vi "数据库插入子vi.vi"(2 "result":string, 3 "2_Leakage":string, 8 "2_Pressure":string, 10 "Serial_No":string) -> ()   [LabVIEW 2014]
panel:
  out "error out":errorcluster
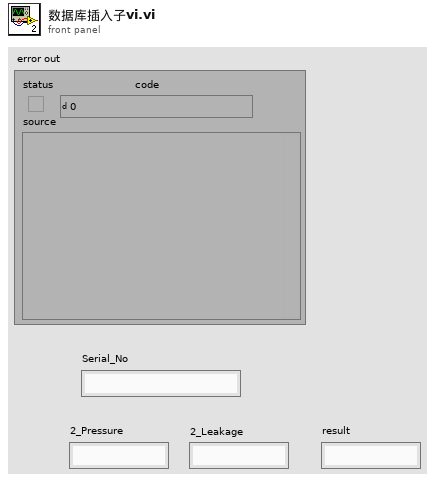
[diagram p1: front panel]
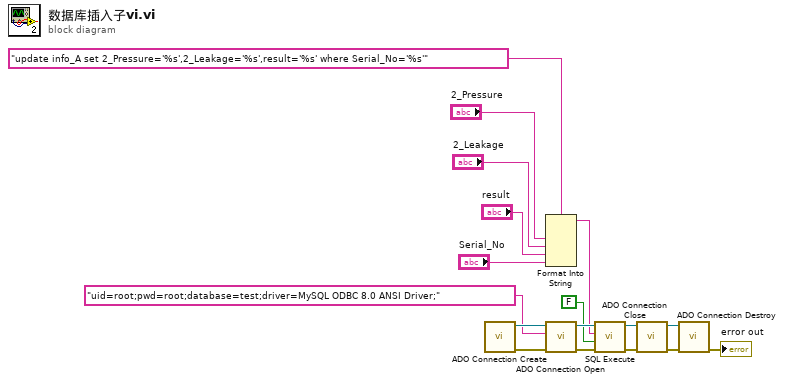
[diagram p0: block diagram]
diagram:
  n1 = call "ADO Connection Create.vi"() -> ("error out"=w16:errorcluster, "ADODB._Connection Out"=w17:refnum<k7>)  [unwired: 10 in]
  n2 = Format Into String(format string="update info_A set 2_Pressure='%s',2_Leakage='%s',result='%s' where Serial_No='%s'" ("Command Text"), "2_Pressure", "2_Leakage", "result", "Serial_No") -> (resulting string=w5:string)  [unwired: 2 in, 1 out]
  n3 = call "ADO Connection Open.vi"("error in (no error)"=w16, "ConnectionString"="uid=root;pwd=root;database=test;driver=MySQL ODBC 8.0 ANSI Driver;", "ADODB._Connection In"=w17) -> ("error out"=w14:errorcluster, "ADODB._Connection Out"=w15:refnum<k7>)  [unwired: 7 in]
  n4 = call "SQL Execute.vi"("error in (no error)"=w14, "Return Data (T)"=FALSE, "Command Text"=w5, "ADODB._Connection In"=w15) -> ("error out"=w12:errorcluster, "ADODB._Connection Out"=w13:refnum<k7>)  [unwired: 4 in, 2 out]
  n5 = call "ADO Connection Close.vi"("error in (no error)"=w12, "ADODB._Connection In"=w13) -> ("error out"=w10:errorcluster, "ADODB._Connection Out"=w11:refnum<k7>)  [unwired: 8 in]
  n6 = call "ADO Connection Destroy.vi"("error in (no error)"=w10, "ADODB._Connection In"=w11) -> ("error out"=→"error out":errorcluster)  [unwired: 9 in]
